vi "PrepareChannels_v2.vi"() -> (0 "DO error out":errorcluster, 1 "DO task out":refnum<k21>, 2 "AO error out":errorcluster, 3 "AO task out":refnum<k21>, 5 "Waveform Graph":waveform(dbl)(graph))   [LabVIEW 2017]
uses:
  <vilib>/DAQmx/configure/timing.llb/DAQmx Timing (Sample Clock).vi
  <vilib>/DAQmx/create/channels.llb/DAQmx Create Channel (AO-Voltage-Basic).vi
  <vilib>/DAQmx/create/channels.llb/DAQmx Create Channel (DO-Digital Output).vi
panel:
  in  "DO Physical channels":tag="pciDAQ/port0/line1:2"
  in  "Sampling Rate (Hz)":dbl=100000.0
  in  "Amplitude (Volts)":dbl=1.0
  in  "Num Pulses":u32=1 min=1
  in  "Pulse Width (ms)":dbl=0.09
  in  "Pulse Type":enum16{"Monophasic", "Biphasic"}(ring)=enum."Biphasic"
  in  "AO Physical channels":tag="pciDAQ/ao0"
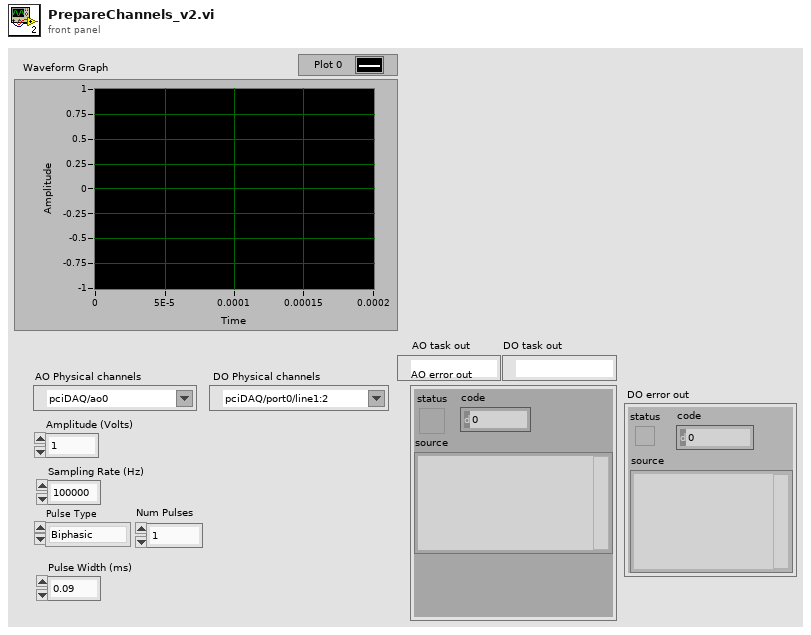
[diagram p1: front panel]
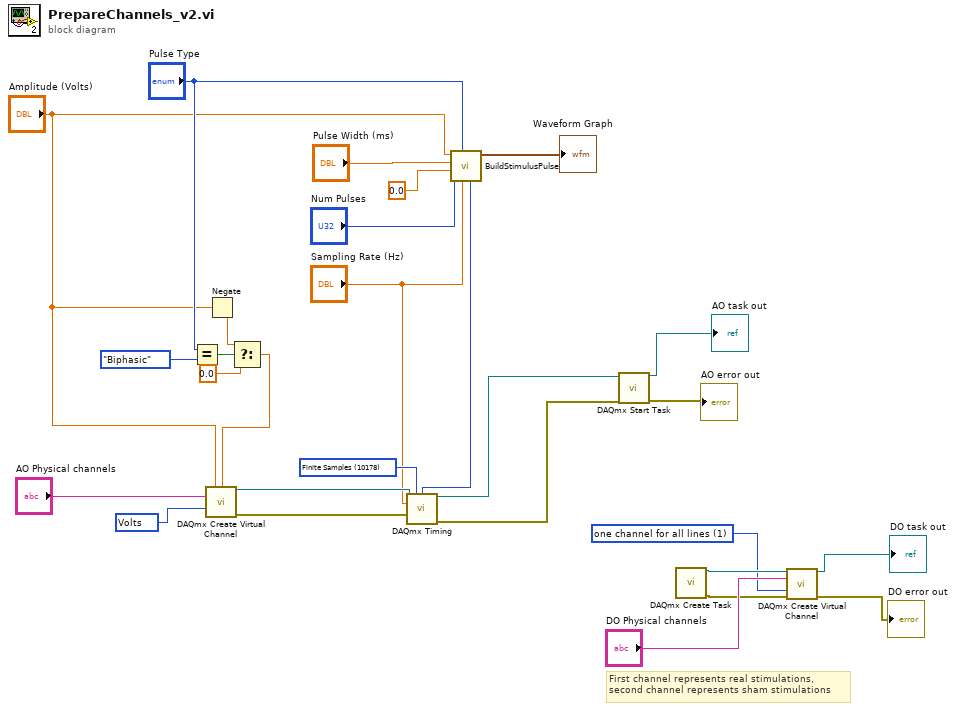
[diagram p0: block diagram]
diagram:
  w1 = 1 items=["one channel for each line", "one channel for all lines"] ("line grouping")
  w23 = 10178 items=["Finite Samples"=10178, "Continuous Samples"=10123, "Hardware Timed Single Point"=12522] ("sample mode")
  w28 = 10348 items=["Volts"=10348, "From Custom Scale"=10065] ("units")
  # "First channel represents real stimulations,\nsecond channel represents sham stimulations"
  n1 = Equal?(x="Pulse Type", y=enum16{"Monophasic", "Biphasic"}."Biphasic") -> (x = y?=w9:bool)
  n2 = Negate(x="Amplitude (Volts)") -> (-x=w7:dbl)
  n3 = Select(t=w7, s=w9, f=0.0) -> (s? t:f=w5:dbl)
  n4 = call-poly <vilib>:"DAQmx Create Virtual Channel.vi"("maximum value"="Amplitude (Volts)", "minimum value"=w5, "physical channels"="AO Physical channels", "units"=w28) -> ("task out"=w22:refnum<k21>, "error out"=w21:errorcluster)  [unwired: 10 in]
  n5 = call "BuildStimulusPulse.vi"("Sampling Rate (Hz)"="Sampling Rate (Hz)", "Pulse Type"="Pulse Type", "Num Pulses"="Num Pulses", "Inter-Pulse Interval (ms)"=0.0, "Pulse Width (ms)"="Pulse Width (ms)", "Amplitude (Volts)"="Amplitude (Volts)") -> ("Waveform Out"=→"Waveform Graph":waveform(dbl), "Final Array Size"=w3:i32)  [unwired: 3 in, 1 out]
  n6 = call-poly <vilib>:"DAQmx Timing.vi"("task/channels in"=w22, "sample mode"=w23, "samples per channel"=w3, "rate"="Sampling Rate (Hz)", "error in"=w21) -> ("task out"=w15:refnum<k21>, "error out"=w14:errorcluster)  [unwired: 9 in]
  n7 = call <vilib>:"DAQmx Start Task.vi"("task/channels in"=w15, "error in"=w14) -> ("task out"=→"AO task out":refnum<k21>, "error out"=→"AO error out":errorcluster)  [unwired: 12 in]
  n8 = call <vilib>:"DAQmx Create Task.vi"() -> ("task out"=w19:refnum<k21>, "error out"=w18:errorcluster)  [unwired: 14 in]
  n9 = call-poly <vilib>:"DAQmx Create Virtual Channel.vi"("task in"=w19, "lines"="DO Physical channels", "line grouping"=w1, "error in"=w18) -> ("task out"=→"DO task out":refnum<k21>, "error out"=→"DO error out":errorcluster)  [unwired: 10 in]
